vi "RSZVB Get Channel Bits.vi"(8 "error in (no error)":errorcluster {"code" format="%.0x"}, 11 "VISA session":refnum<visa-resource-name>) -> (0 "error out":errorcluster {"code" format="%.0x"}, 2 "Channel Bits":i32, 3 "dup VISA session":refnum<visa-resource-name>)   [LabVIEW 2011]
doc: "This VI queries a channel-dependent four-bit decimal value to control four independent output signals at the USER CONTROL connector (applied to pins 8, 9, 10, 11). The output signals are 3.3 V TTL signals which can be used to differentiate between up to 16 independent analyzer states. This VI itself does not change the analyzer state.\n\nRemote-control command(s):\nCONTrol:AUXiliary:C[:DATA]?"
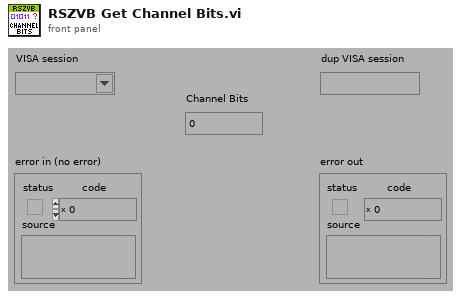
[diagram p1: front panel]
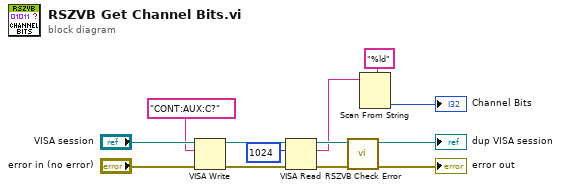
[diagram p0: block diagram]
diagram:
  n1 = VISA Write(VISA resource name="VISA session", write buffer="CONT:AUX:C?", error in (no error)="error in (no error)") -> (VISA resource name out=w11:refnum<visa-resource-name>, error out=w13:errorcluster)  [unwired: 1 out]
  n2 = VISA Read(VISA resource name=w11, byte count=u32 1024 ("byte count (0)"), error in (no error)=w13) -> (VISA resource name out=w10:refnum<visa-resource-name>, read buffer=w7:string, error out=w9:errorcluster)  [unwired: 1 out]
  n3 = call "RSZVB Check Error.vi"("error in (no error)"=w9, "VISA session"=w10) -> ("error out"=→"error out":errorcluster, "dup VISA session"=→"dup VISA session":refnum<visa-resource-name>)  [unwired: 8 in]
  n4 = Scan From String(format string="%ld", input string=w7) -> (output 1=→"Channel Bits":i32)  [unwired: 3 in, 3 out]
